vi "ZaberSimpleCommand.vi"(0 "VISA Refnum in":refnum<visa-resource-name>, 5 "Num1":i32, 7 "Cmd":i32, 9 "Val":i32, 11 "Resp num":i32) -> (6 "Num1":u8, 8 "Cmd":u8, 10 "Val":i32)   [LabVIEW 2013]
uses:
  <instrlib>/ZaberTSeries/ZaberTSeries.lvlib
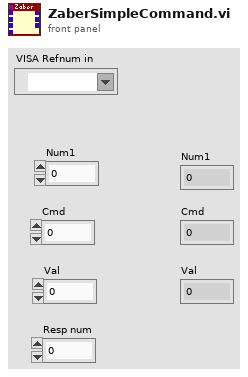
[diagram p1: front panel]
types:
  T1 = cluster{"Num1":i32, "Cmd":i32, "Val":i32, "Resp num":i32}
  T2 = typedef "ZaberTSeries.lvlib/Response.ctl" = cluster{"Device Number":u8, "Command":u8, "Data":i32}
  T3 = cluster{"Responses out[0]":T2, "Responses out[1]":T2, "Responses out[2]":T2, "Responses out[3]":T2, "Responses out[4]":T2, "Responses out[5]":T2, "Responses out[6]":T2, "Responses out[7]":T2, "Responses out[8]":T2}
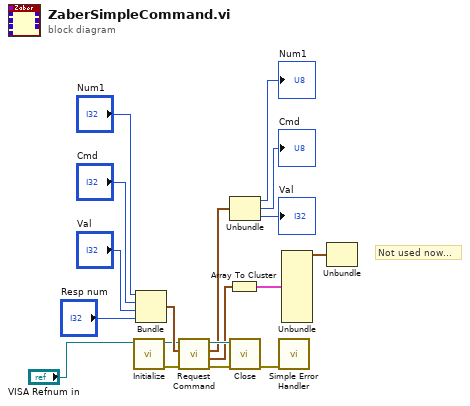
[diagram p0: block diagram]
diagram:
  # "Not used now..."
  n1 = call <instrlib>:"Initialize.vi"("VISA resource name"="VISA Refnum in") -> ("error out"=w2:errorcluster, "VISA resource name out"=w1:refnum<visa-resource-name>)  [unwired: 8 in, 1 out]
  n2 = Bundle("Num1"="Num1", "Cmd"="Cmd", "Val"="Val", "Resp num"="Resp num") -> (w11:T1)  [unwired: 1 in]
  n3 = call <instrlib>:"Request Command.vi"("error in (no error)"=w2, "Request"=w11, "VISA resource name"=w1) -> ("error out"=w12:errorcluster, "Responses out"=w10:T2[], "First Response"=w7:T2, "VISA resource name out"=w13:refnum<visa-resource-name>)  [unwired: 5 in]
  n4 = Array To Cluster(array=w10) -> (cluster=w9:T3)
  n5 = Unbundle(w7) -> ("Device Number"=→"Num1":u8, "Command"=→"Cmd":u8, "Data"=→"Val":i32)
  n6 = call <instrlib>:"Close.vi"("error in (no error)"=w12, "VISA resource name"=w13) -> ("error out"=w14:errorcluster)  [unwired: 8 in, 1 out]
  n7 = call <vilib>:"Simple Error Handler.vi"("error in (no error)"=w14) -> ()  [unwired: 4 in, 5 out]
  n8 = Unbundle(w9) -> ("Responses out[0]"=w8:T2)  [unwired: 8 out]
  n9 = Unbundle(w8) -> ()  [unwired: 3 out]
